vi "Configure Timebase.vi"(7 "Record Length (10k points)":u32(ring)=10000 items=["1k"=1000, "10k"=10000, "100k"=100000], 8 "error in (no error)":errorcluster, 9 "Position (0.0 s)":dbl, 10 "Time per Division (0.0005 s)":dbl=0.0005, 11 "VISA resource name":refnum<visa-resource-name>) -> (0 "error out":errorcluster, 3 "VISA resource name out":refnum<visa-resource-name>)   [LabVIEW 2013, in "Template - Scope.lvlib"]
doc: "Configures the timebase and horizontal features of the oscilloscope."
uses:
  <instrlib>/_Template - Scope/Template - Scope.lvlib
panel:
  # "EDIT: Update the ring control with the appropriate values for your instrument. If the instrument does not support a predefined list of values, replace the ring control with the numeric control."
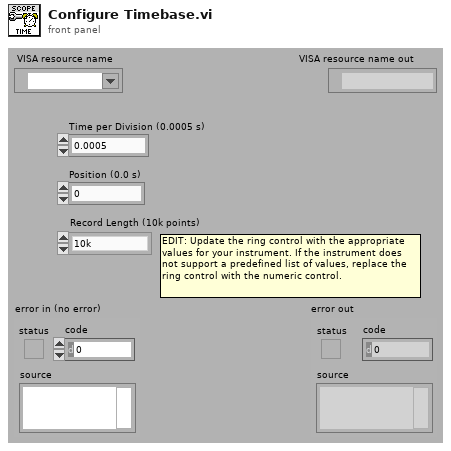
[diagram p1: front panel]
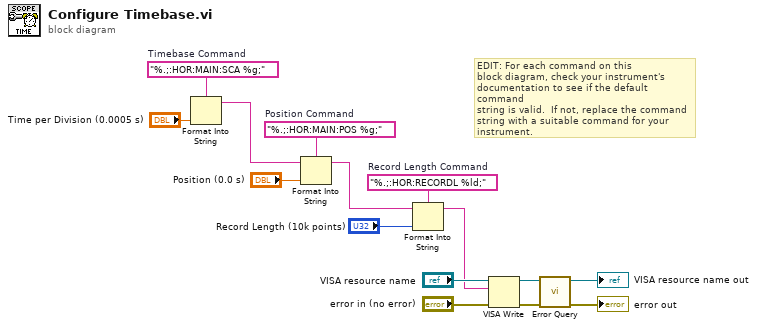
[diagram p0: block diagram]
diagram:
  w1 = "%.;:HOR:RECORDL %ld;"  # Record Length Command
  w7 = "%.;:HOR:MAIN:POS %g;"  # Position Command
  w9 = "%.;:HOR:MAIN:SCA %g;"  # Timebase Command
  # "EDIT: For each command on this\nblock diagram, check your instrument's\ndocumentation to see if the default command\nstring is valid.  If not, replace the command\nstring with a suitable command for your\ninstrument."
  n1 = Format Into String(format string=w9, "Time per Division (0.0005 s)") -> (resulting string=w6:string)  [unwired: 2 in, 1 out]
  n2 = Format Into String(format string=w7, initial string=w6, "Position (0.0 s)") -> (resulting string=w4:string)  [unwired: 1 in, 1 out]
  n3 = Format Into String(format string=w1, initial string=w4, "Record Length (10k points)") -> (resulting string=w3:string)  [unwired: 1 in, 1 out]
  n4 = VISA Write(VISA resource name="VISA resource name", write buffer=w3, error in (no error)="error in (no error)") -> (VISA resource name out=w11:refnum<visa-resource-name>, error out=w10:errorcluster)  [unwired: 1 out]
  n5 = call <instrlib>:"Error Query.vi"("error in (no error)"=w10, "VISA resource name"=w11) -> ("error out"=→"error out":errorcluster, "VISA resource name out"=→"VISA resource name out":refnum<visa-resource-name>)  [unwired: 6 in, 2 out]
